vi "Write Clocks.vi"(8 "error in (no error)":errorcluster, 10 "Clocks":T1[](array[typedef]), 11 "NiPxi6683H in":refnum<class "NiPxi6683H.lvclass">) -> (0 "error out":errorcluster, 3 "NiPxi6683H out":refnum<class "NiPxi6683H.lvclass">)   [LabVIEW 2014, in "SyncPlugins.lvlib" / "NiPxi6683H.lvclass"]
uses:
  NiPxi6683H.lvclass
  PXI_MultiTrig/Typedefs/clClocks.ctl
  NiPxi6683H.lvclass/NiPxi6683H.ctl
  PXI_MultiTrig/PXI_MultiTrig.lvclass
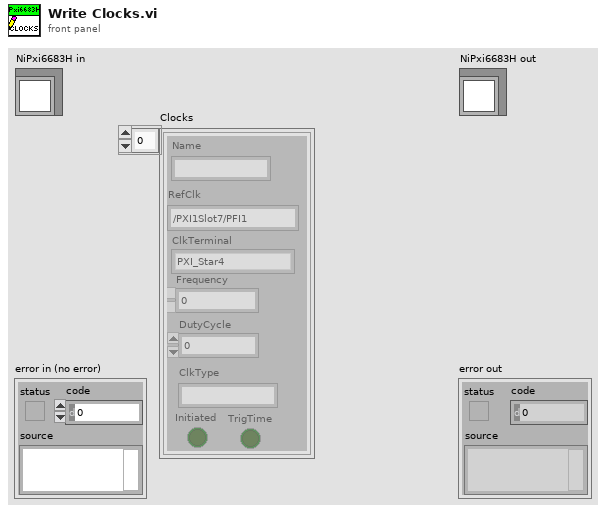
[diagram p1: front panel]
types:
  T1 = typedef "SyncPlugins.lvlib/PXI_MultiTrig.lvclass/clClocks.ctl" = cluster{"Name":string, "RefClk":string, "ClkTerminal":string, "Frequency":dbl, "DutyCycle":dbl, "ClkType":string, "Initiated":bool, "TrigTime":bool}
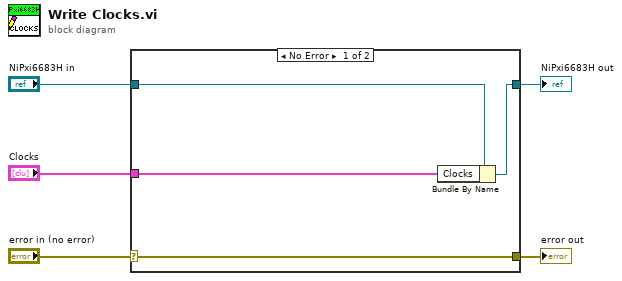
[diagram p0: block diagram]
diagram:
  n1 = case shown="No Error" "error in (no error)" {
    selector: "error in (no error)" -> [w9 w10]
    tunnel: [w9 w10] -> w4
    tunnel: [w7 w11] -> w2
    tunnel: "NiPxi6683H in" -> [w8 w11]
    tunnel: "Clocks" -> [w6 _]
    frame No Error {
      n2 = Bundle By Name(cluster=w8, "Clocks"=w6) -> (w7:refnum<class "NiPxi6683H.lvclass">)
    }
    frame Error {
    }
  }
  "error out" <- w4
  "NiPxi6683H out" <- w2
